vi "Lab1_1.vi"() -> ()   [LabVIEW 2021]
panel:
  out "Numeric 2":dbl
  out "Numeric":dbl
  in  "stop":bool
  in  "Temperature (F)":dbl(slide) scale=0.0..100.0
  out "Temperature (C)":dbl(slide) scale=0.0..100.0
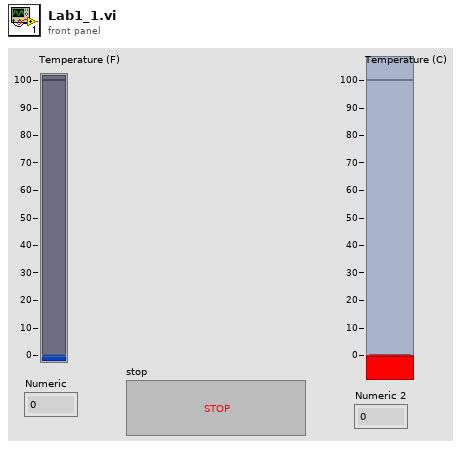
[diagram p1: front panel]
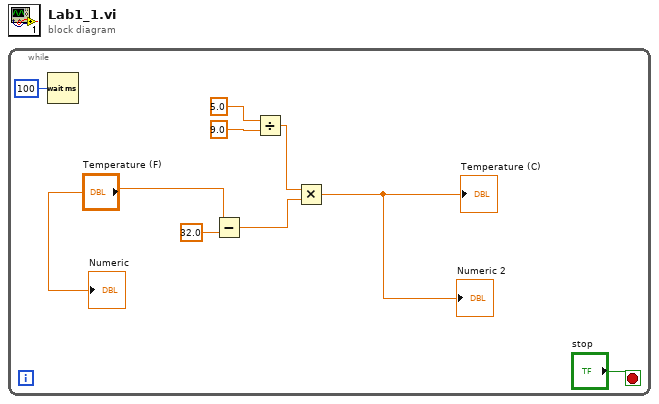
[diagram p0: block diagram]
diagram:
  n1 = while {
    stop <- "stop" stop-if-true
    n2 = Wait (ms)(milliseconds to wait=u32 100) -> ()  [unwired: 1 out]
    n3 = Subtract(x="Temperature (F)", y=32.0) -> (x-y=w9:dbl)
    n4 = Divide(x=5.0, y=9.0) -> (x/y=w8:dbl)
    n5 = Multiply(x=w8, y=w9) -> (x*y=→"Temperature (C)" →"Numeric 2":dbl)
    "Numeric" <- "Temperature (F)"
  }
